vi "main1.vi"() -> (0 "error out":errorcluster)   [LabVIEW 2012]
uses:
  <vilib>/Utility/file.llb/Read From Spreadsheet File (string).vi
  Global1.vi
panel:
  out "element 2":string
  out "error out 2":errorcluster
  out "standard error 4":string
  out "element":string
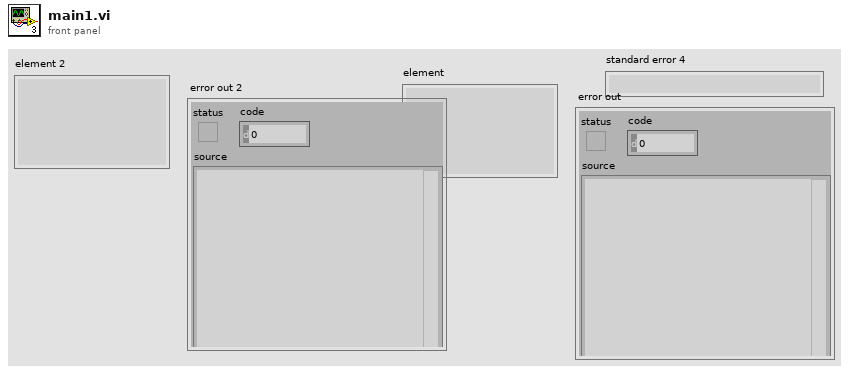
[diagram p1: front panel]
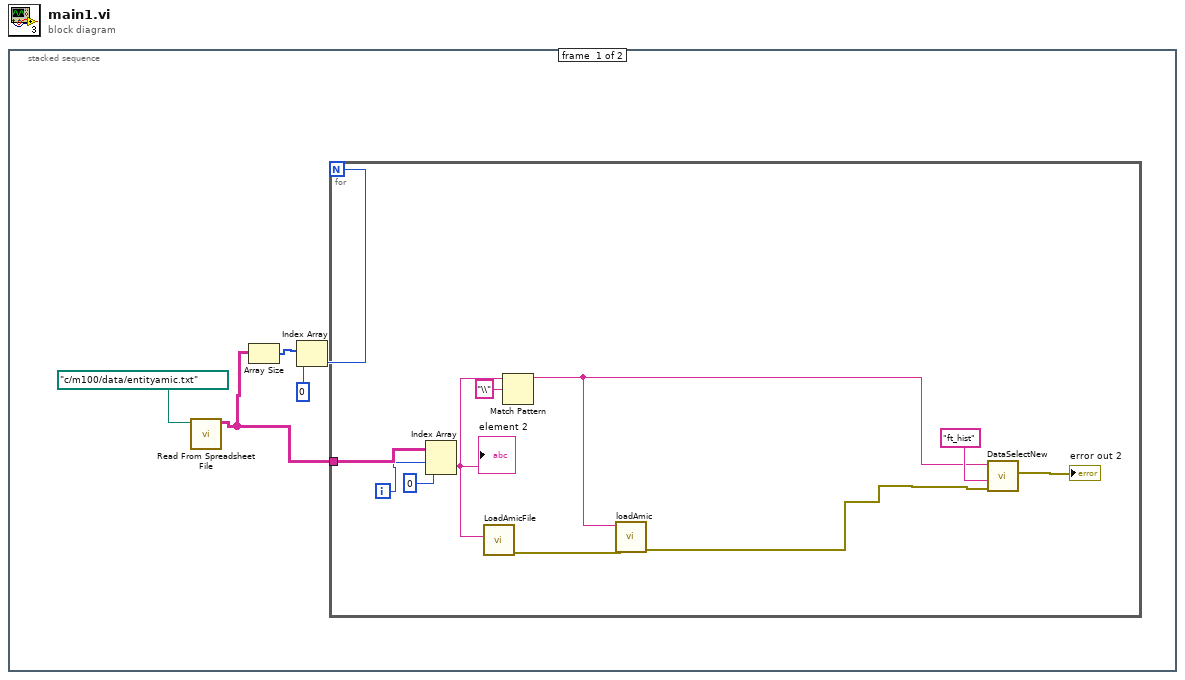
[diagram p0: block diagram]
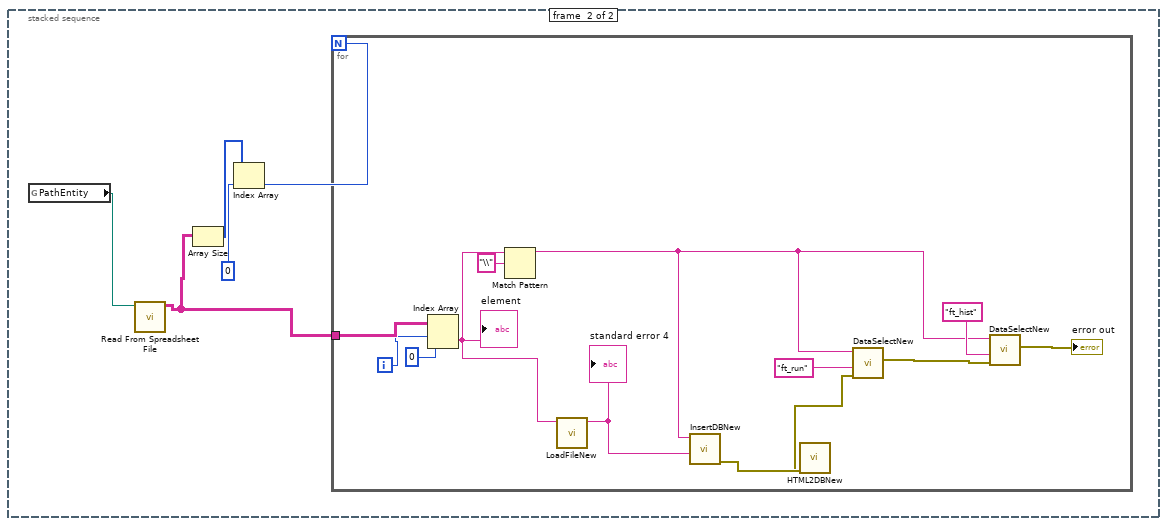
[diagram p2: hidden frame]
diagram:
  n1 = stacked-sequence {
    frame #0 {
      n2 = call-poly <vilib>:"Read From Spreadsheet File.vi"("file path (dialog if empty)"=path "c:/m100/data/entityamic.txt" ("file path (use dialog)")) -> ("all rows"=w1:string[][])  [unwired: 6 in, 4 out]
      n3 = Array Size(array=w1) -> (size(s)=w4:i32[])
      n4 = Index Array(array=w4, index=0) -> (element=w2:i32)
      n5 = for {
        N: w2 -> [_]
        tunnel: w1 -> [w15]
        i -> [w13]
        n6 = Index Array(array=w15, index (row)=w13, index (col)=0 ("disabled index (col)")) -> (element=w9:string)
        "element 2" <- w9
        n7 = call "LoadAmicFile.vi"("folder"=w9) -> ("error out"=w8:errorcluster)  [unwired: 9 in, 1 out]
        n8 = Match Pattern(string=w9, regular expression="\\") -> (before substring=w7:string)  [unwired: 1 in, 3 out]
        n9 = call "loadAmic.vi"("error in"=w8, "machine"=w7) -> ("error out"=w6:errorcluster)  [unwired: 9 in]
        n10 = call "DataSelectNew.vi"("error in (no error)"=w6, "Table"="ft_hist", "Machine"=w7) -> ("error out"=→"error out 2":errorcluster)  [unwired: 8 in]
      }
    }
    frame #1 {
      n11 = global read "Global1.vi" "PathEntity"() -> (w16:path)
      n12 = call-poly <vilib>:"Read From Spreadsheet File.vi"("file path (dialog if empty)"=w16) -> ("all rows"=w17:string[][])  [unwired: 6 in, 4 out]
      n13 = Array Size(array=w17) -> (size(s)=w20:i32[])
      n14 = Index Array(array=w20, index=0) -> (element=w18:i32)
      n15 = for {
        N: w18 -> [_]
        tunnel: w17 -> [w33]
        i -> [w31]
        n16 = Index Array(array=w33, index (row)=w31, index (col)=0 ("disabled index (col)")) -> (element=w29:string)
        "element" <- w29
        n17 = Match Pattern(string=w29, regular expression="\\") -> (before substring=w21:string)  [unwired: 1 in, 3 out]
        n18 = call "LoadFileNew.vi"("folder"=w29) -> ("Lot"=w24:string)  [unwired: 9 in, 1 out]
        "standard error 4" <- w24
        n19 = call "InsertDBNew.vi"("String"=w24, "Entity"=w21) -> ("error out"=w23:errorcluster)  [unwired: 9 in]
        n20 = call "HTML2DBNew.vi"("error in (no error)"=w23) -> ("error out"=w22:errorcluster)  [unwired: 10 in]
        n21 = call "DataSelectNew.vi"("error in (no error)"=w22, "Table"="ft_run", "Machine"=w21) -> ("error out"=w27:errorcluster)  [unwired: 8 in]
        n22 = call "DataSelectNew.vi"("error in (no error)"=w27, "Table"="ft_hist", "Machine"=w21) -> ("error out"=→"error out":errorcluster)  [unwired: 8 in]
      }
    }
  }
